vi "Select channel.vi"(7 "Channel Info":T1(array[cluster]) {"sensor sensitivity (mV/EU)" format="%.2f"; "offset" format="%.2f"; "multiplier" format="%.2f"}) -> (2 "index":i32, 3 "channel name":string)   [LabVIEW 2017]
panel:
  in  "OK":bool
  in  "Channel List":i32(listbox)
  # "Select channel from list"
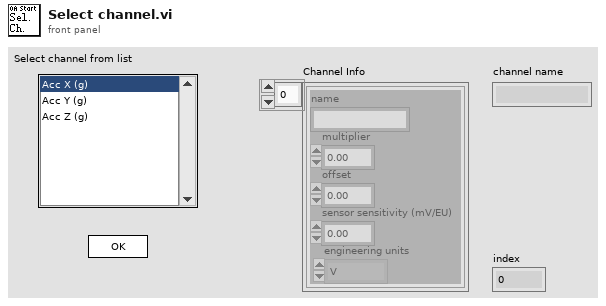
[diagram p1: front panel]
types:
  T1 = cluster{"name":string, "multiplier":sgl, "offset":sgl, "sensor sensitivity (mV/EU)":dbl, "engineering units":enum16{"custom...", "V", "Pa", "g", "m/s^2", "m/s", "m", "in/s^2", "in/s", "in"}}[]
  T2 = enum16{"custom...", "V", "Pa", "g", "m/s^2", "m/s", "m", "in/s^2", "in/s", "in"}
  T3 = cluster{"name":string, "multiplier":sgl, "offset":sgl, "sensor sensitivity (mV/EU)":dbl, "engineering units":enum16{"custom...", "V", "Pa", "g", "m/s^2", "m/s", "m", "in/s^2", "in/s", "in"}}
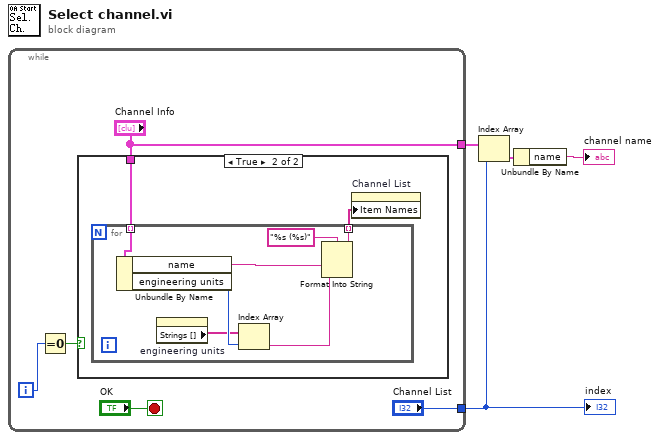
[diagram p0: block diagram]
diagram:
  n1 = while {
    tunnel: ["Channel Info"] -> w4
    tunnel: ["Channel List"] -> w3
    i -> [w9]
    stop <- "OK" stop-if-true
    n2 = Equal To 0?(x=w9) -> (x = 0?=w8:bool)
    n3 = case shown="True" w8 {
      tunnel: "Channel Info" -> [_ w10]
      frame False {
      }
      frame True {
        n4 = for {
          tunnel: w10 -> [w18] mode=indexing
          tunnel: [w13] -> w11 mode=indexing
          n5 = Unbundle By Name(w18) -> ("name"=w15:string, "engineering units"=w17:T2)
          n6 = property on="engineering units" class="Enum (strict)"() -> ("Strings []"=w16:string[])  [unwired: 2 in, 2 out]
          n7 = Index Array(array=w16, index=w17) -> (element=w14:string)
          n8 = Format Into String(format string="%s (%s)" ("Input String"), w15, w14) -> (resulting string=w13:string)  [unwired: 2 in, 1 out]
        }
        n9 = property on="Channel List" class="LstBox (strict)"("Item Names"=w11) -> ()  [unwired: 2 in, 2 out]
      }
    }
  }
  "index" <- w3
  n10 = Index Array(array=w4, index=w3) -> (element=w2:T3)
  n11 = Unbundle By Name(w2) -> ("name"=→"channel name":string)
